vi "Step.vi"(8 "error in":errorcluster, 10 "Up?":bool, 11 "Stepper.lvclass":refnum<class "Stepper.lvclass">) -> (0 "error out":errorcluster, 1 "Coil Status":bool[](array[boolean]), 3 "Stepper.lvclass out":refnum<class "Stepper.lvclass">)   [LabVIEW 2012, in "Stepper.lvclass"]
uses:
  Stepper.lvclass
  Stepper.lvclass/Stepper.ctl
  <vilib>/DAQmx/write.llb/DAQmx Write (Digital 1D Bool 1Chan 1Samp).vi
  <vilib>/DAQmx/miscellaneous.llb/DAQmx Fill In Error Info.vi
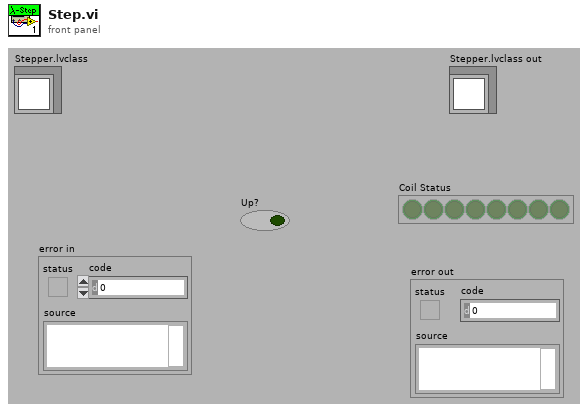
[diagram p1: front panel]
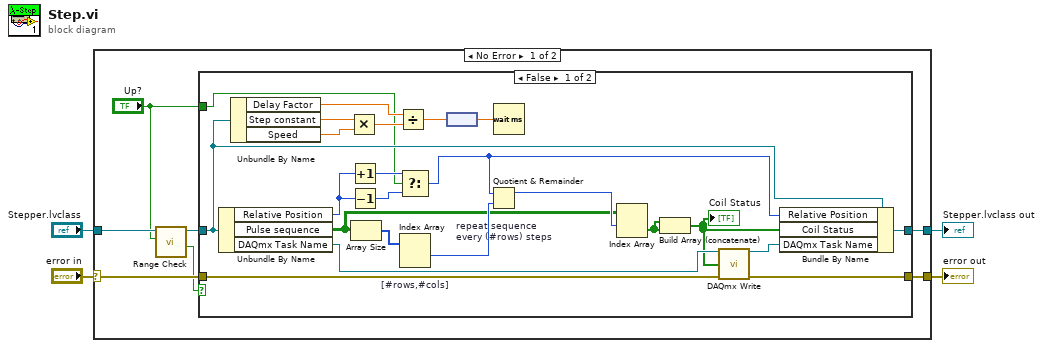
[diagram p0: block diagram]
diagram:
  n1 = case shown="No Error" "error in" {
    selector: "error in" -> [w10 w38]
    tunnel: "Stepper.lvclass" -> [w8 w37]
    tunnel: [w11 w37] -> w3
    tunnel: [w9 w38] -> w1
    frame No Error {
      n2 = call "Range Check.vi"("Direction"="Up?", "Stepper.lvclass"=w8) -> ("Out of range?"=w6:bool, "Stepper.lvclass out"=w7:refnum<class "Stepper.lvclass">)  [unwired: 8 out]
      n3 = case shown="False" w6 {
        tunnel: [w29 w36] -> w11
        tunnel: w10 -> [w25 w35]
        tunnel: [w24 w35] -> w9
        tunnel: w7 -> [w20 w36]
        tunnel: "Up?" -> [w12 _]
        frame False {
          n4 = Unbundle By Name(w20) -> ("Relative Position"=w28:i32, "Pulse sequence"=w23:bool[][], "DAQmx Task Name"=w22:refnum<k21>)
          n5 = Unbundle By Name(w20) -> ("Delay Factor"=w18:dbl, "Step constant"=w15:dbl[unit], "Speed"=w17:dbl[unit])
          n6 = Multiply(x=w15, y=w17) -> (x*y=w19:dbl[unit])
          n7 = Increment(x=w28) -> (x+1=w31:i32)
          n8 = Decrement(x=w28) -> (x-1=w32:i32)
          n9 = Array Size(array=w23) -> (size(s)=w33:i32[])
          n10 = Divide(x=w18, y=w19) -> (x/y=w16:dbl[unit])
          n11 = Select(t=w31, s=w12, f=w32) -> (s? t:f=w27:i32)
          n12 = Index Array "[#rows,#cols]"(array=w33) -> (element #1=w34:i32)  [unwired: 2 in, 1 out]
          n13 = node(w16) -> (w14:dbl)
          n14 = Quotient & Remainder "repeat sequence\nevery (#rows) steps"(x=w27, y=w34) -> (x-y*floor(x/y)=w26:i32)  [unwired: 1 out]
          n15 = Wait (ms)(milliseconds to wait=w14) -> ()  [unwired: 1 out]
          n16 = Index Array(array=w23, index (row)=w26) -> (element=w30:bool[])  [unwired: 1 in]
          n17 = Build Array (concatenate)(w30, w30) -> (w13:bool[])
          "Coil Status" <- w13
          n18 = call-poly <vilib>:"DAQmx Write.vi"("task/channels in"=w22, "data"=w13, "error in"=w25) -> ("task out"=w21:refnum<k21>, "error out"=w24:errorcluster)  [unwired: 1 in, 10 out]
          n19 = Bundle By Name(cluster=w20, "Relative Position"=w27, "Coil Status"=w13, "DAQmx Task Name"=w21) -> (w29:refnum<class "Stepper.lvclass">)
        }
        frame True {
        }
      }
    }
    frame Error {
    }
  }
  "Stepper.lvclass out" <- w3
  "error out" <- w1
